vi "Add Children to Tree.vi"(8 "error in (no error)":errorcluster, 9 "Parent Tag":string, 10 "Tree Manager in":refnum<class "Tree Manager.lvclass">, 11 "Data Item in":refnum<class "Data Item.lvclass">) -> (0 "error out":errorcluster, 2 "Tree Manager out":refnum<class "Tree Manager.lvclass">, 3 "Data Item out":refnum<class "Data Item.lvclass">)   [LabVIEW 2026, in "VILab.lvlib" / "Data Item.lvclass"]
uses:
  Data Item.lvclass
  Tree Manager/Tree Manager.lvclass
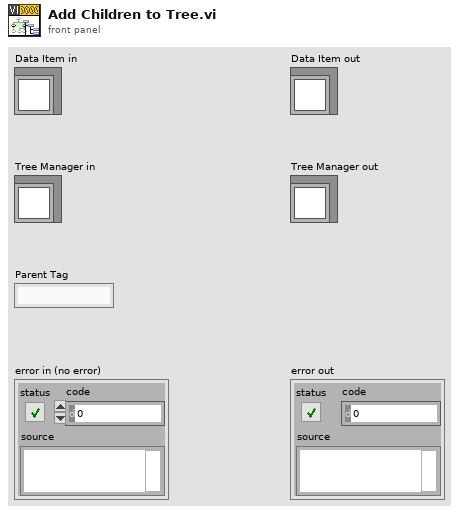
[diagram p1: front panel]
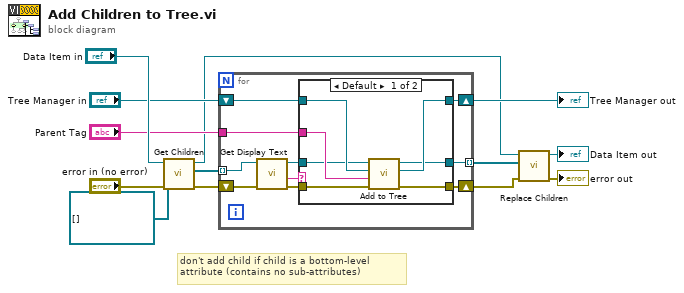
[diagram p0: block diagram]
diagram:
  # "don't add child if child is a bottom-level attribute (contains no sub-attributes)"
  n1 = call-dynamic "Get Children.vi"("error in (no error)"="error in (no error)", "All Data"=refnum<class "Data Item.lvclass">[] [], "Data Item in"="Data Item in") -> ("error out"=w12:errorcluster, "Children"=w13:refnum<class "Data Item.lvclass">[], "Data Item out"=w2:refnum<class "Data Item.lvclass">)  [unwired: 5 in, 1 out]
  n2 = for {
    shift-right: [w20] -> w5
    shift-left: "Tree Manager in" -> [w22]
    shift-right: [w21] -> w8
    shift-left: w12 -> [w15]
    tunnel: w13 -> [w23] mode=indexing
    tunnel: "Parent Tag" -> [w19]
    tunnel: [w18] -> w6 mode=indexing
    n3 = call-dynamic "Get Display Text.vi"("error in (no error)"=w15, "Data Item in"=w23) -> ("error out"=w14:errorcluster, "Detail Text"=w16:string, "Data Item out"=w17:refnum<class "Data Item.lvclass">)  [unwired: 6 in, 1 out]
    n4 = case shown="Default" w16 {
      tunnel: w22 -> [w30 w33]
      tunnel: w14 -> [w29 w31]
      tunnel: [w28 w31] -> w21
      tunnel: [w27 w33] -> w20
      tunnel: w19 -> [w26 _]
      tunnel: [w25 w32] -> w18
      tunnel: w17 -> [w24 w32]
      frame Default {
        n5 = call-dynamic "Add to Tree.vi"("error in (no error)"=w29, "Parent Tag"=w26, "Tree Manager in"=w30, "Data Item in"=w24) -> ("error out"=w28:errorcluster, "Tree Manager out"=w27:refnum<class "Tree Manager.lvclass">, "Data Item out"=w25:refnum<class "Data Item.lvclass">)  [unwired: 5 in]
      }
      frame "" {
      }
    }
  }
  "Tree Manager out" <- w5
  n6 = call-dynamic "Replace Children.vi"("error in (no error)"=w8, "New Children"=w6, "Data Item in"=w2) -> ("error out"=→"error out":errorcluster, "Data Item out"=→"Data Item out":refnum<class "Data Item.lvclass">)  [unwired: 7 in]
